vi "Tango Data Position.vi"(7 "XYZ notifier":refnum<notifier>, 8 "error in (no error)":errorcluster, 11 "Hardware Resources in":T1={"Tango HW"={"VISA resource"="", "Baud Rate (115200)"=2, "lAnInterfaceType"=0, "bAShowProt"=15}, "Writer Queue"=refnum, "Status"=FALSE, "Abs Position"=[], "Axis Velocity"={"dX"=0.0, "dY"=0.0, "dZ"=0.0, "dA"=0.0}, "acceleration "=0.0, "Z direction"=enum."Up", "Position Mode"="", "plLSID"=0}) -> (0 "error out":errorcluster, 2 "Message Data Out":variant, 3 "Hardware Resources out":T1={"Tango HW"={"VISA resource"="", "Baud Rate (115200)"=2, "lAnInterfaceType"=0, "bAShowProt"=15}, "Writer Queue"=refnum, "Status"=FALSE, "Abs Position"=[], "Axis Velocity"={"dX"=0.0, "dY"=0.0, "dZ"=0.0, "dA"=0.0}, "acceleration "=0.0, "Z direction"=enum."Up", "Position Mode"="", "plLSID"=0})   [LabVIEW 2020, in "MOTOR.lvlib"]
doc: "Generates sample waveforms according to the signal type in the HW Config input."
uses:
  MOTOR.lvlib
  PS Hardware Configuration.ctl
  support/Message Queue/Message Cluster.ctl
  support/PCT FGV CMD.ctl
  <instrlib>/Tango_DLL/Tango_DLL.lvlib
  support/Message Queue/Message Queue.lvlib
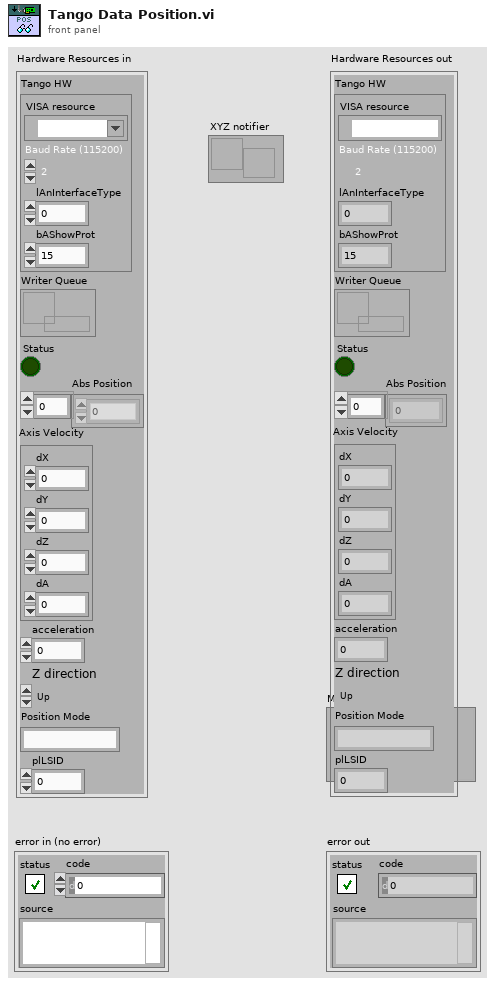
[diagram p1: front panel]
types:
  T1 = typedef "MOTOR.lvlib/PS Hardware Configuration.ctl" = cluster{"Tango HW":cluster{"VISA resource":refnum<visa-resource-name>, "Baud Rate (115200)":i32, "lAnInterfaceType":i32, "bAShowProt":i32}, "Writer Queue":refnum<queue>, "Status":bool, "Abs Position":i32[], "Axis Velocity":cluster{"dX":dbl, "dY":dbl, "dZ":dbl, "dA":dbl}, "acceleration ":dbl, "Z direction":enum16{"Up", "Down"}, "Position Mode":string, "plLSID":i32}
  T2 = typedef "PCT FGV CMD.ctl" = enum16{"INIT", "GET", "SET"}
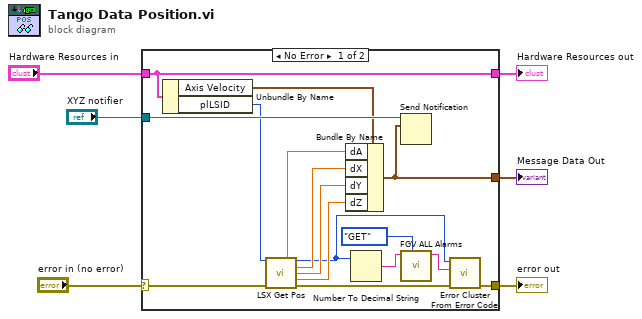
[diagram p0: block diagram]
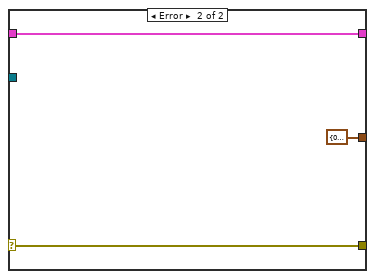
[diagram p2: hidden frame]
diagram:
  n1 = case shown="No Error" "error in (no error)" {
    selector: "error in (no error)" -> [w9 w25]
    tunnel: [w18 w25] -> w5
    tunnel: [w19 cluster{"dX":dbl, "dY":dbl, "dZ":dbl, "dA":dbl} {"dX"=0.0, "dY"=0.0, "dZ"=0.0, "dA"=0.0} ("output cluster")] -> w4
    tunnel: "Hardware Resources in" -> [w21 w24]
    tunnel: [w21 w24] -> w2
    tunnel: "XYZ notifier" -> [w22 _]
    frame No Error {
      n2 = Unbundle By Name(w21) -> ("Axis Velocity"=w20:cluster{"dX":dbl, "dY":dbl, "dZ":dbl, "dA":dbl}, "plLSID"=w14:i32)
      n3 = call <instrlib>:"LSX Get Pos.vi"("lLSID"=w14, "error in (no error)"=w9) -> ("pdA out"=w13:dbl, "function return"=w7:i32, "pdX out"=w12:dbl, "pdY out"=w11:dbl, "pdZ out"=w10:dbl, "error out"=w8:errorcluster)  [unwired: 8 in]
      n4 = Bundle By Name(cluster=w20, "dA"=w13, "dX"=w12, "dY"=w11, "dZ"=w10) -> (w19:cluster{"dX":dbl, "dY":dbl, "dZ":dbl, "dA":dbl})
      n5 = Number To Decimal String(number=w7) -> (decimal integer string=w16:string)  [unwired: 1 in]
      n6 = Send Notification(notification=w19, notifier=w22) -> ()  [unwired: 1 in, 2 out]
      n7 = call "FGV ALL Alarms.vi"("CMD"=PCT_FGV_CMD."GET", "name"=w16) -> ("Alarm MSG out"=w15:string)  [unwired: 8 in, 1 out]
      n8 = call <vilib>:"Error Cluster From Error Code.vi"("error in (no error)"=w8, "error message (\"\")"=w15, "error code (0)"=w7) -> ("error out"=w18:errorcluster)  [unwired: 6 in]
    }
    frame Error {
    }
  }
  "error out" <- w5
  "Message Data Out" <- w4
  "Hardware Resources out" <- w2
